vi "Write Limits File.vi"(0 "Limits File Path":path, 5 "Limit Data":T1, 11 "error in (no error)":errorcluster) -> (15 "error out":errorcluster)   [LabVIEW 2020]
doc: "Write Limit File writes the waveform data to the Limit file."
uses:
  Plot Data.ctl
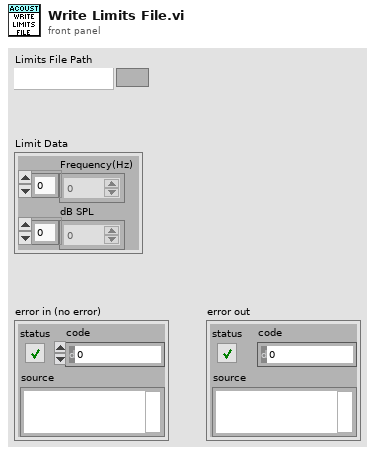
[diagram p1: front panel]
types:
  T1 = typedef "Plot Data.ctl" = cluster{"Frequency(Hz)":dbl[], "dB SPL":dbl[]}
  T2 = enum16{"open", "replace", "create", "open or create", "replace or create", "replace or create with confirmation"}
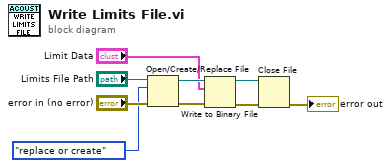
[diagram p0: block diagram]
diagram:
  n1 = Open/Create/Replace File(file path (use dialog)="Limits File Path", error in="error in (no error)", operation (0:open)=T2."replace or create") -> (refnum out=w7:refnum<file>, error out=w6:errorcluster)  [unwired: 3 in, 1 out]
  n2 = Write to Binary File(file (use dialog)=w7, data="Limit Data", error in=w6) -> (refnum out=w3:refnum<file>, error out=w4:errorcluster)  [unwired: 3 in, 1 out]
  n3 = Close File(refnum=w3, error in=w4) -> (error out=→"error out":errorcluster)  [unwired: 1 out]
